vi "cRIO_FPGA_COMMUNICATION Schreibe Ausgangsdaten.vi"(8 "error in (no error)":errorcluster caption="Fehler (Eingang, kein Fehler)", 9 "Station":bool[](array[boolean])=[FALSE, FALSE, FALSE, FALSE, FALSE, FALSE, FALSE, FALSE], 10 "Band":bool[](array[boolean])=[FALSE, FALSE, FALSE, FALSE, FALSE, FALSE, FALSE, FALSE], 11 "Station Index":T1) -> (0 "error out":errorcluster caption="Fehler (Ausgang)")   [LabVIEW 2013, in "cRIO_FPGA_COMMUNICATION.lvlib"]
uses:
  cRIO_FPGA_COMMUNICATION.lvlib
  TYPES/TYPE Station Index.ctl
  TYPES/TYPE Band und Stations Kommandos.ctl
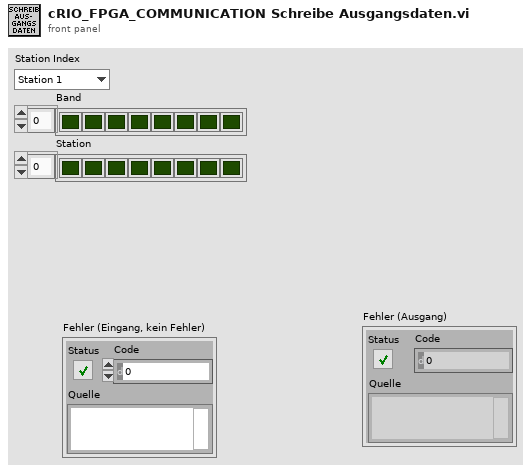
[diagram p1: front panel]
types:
  T1 = typedef "cRIO_FPGA_COMMUNICATION.lvlib/TYPE Station Index.ctl" = enum16{"Station 1", "Station 2", "Station 3", "Station 4", "Station 5", "Station 6", "Station 7", "Station 8", "Station 9", "Station 10", "Station 11", "Station 12", "Station 13", "Station 14", "Station 15", "Station 16", "Station 17", "Station 18", "Station 19", "Station 20"}
  T2 = typedef "cRIO_FPGA_COMMUNICATION.lvlib/TYPE Band und Stations Kommandos.ctl" = enum16{"Init", "Lese", "Schreibe"}
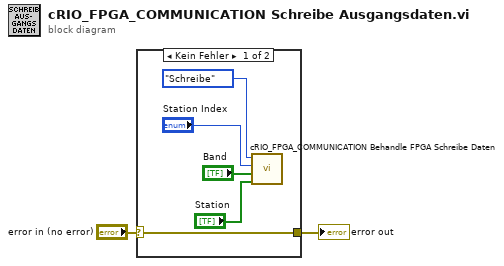
[diagram p0: block diagram]
diagram:
  n1 = case shown="Kein Fehler" "error in (no error)" {
    selector: "error in (no error)" -> [w7 w8]
    tunnel: [w7 w8] -> w1
    frame No Error {
      n2 = call "cRIO_FPGA_COMMUNICATION Behandle FPGA Schreibe Daten.vi"("Station"="Station", "Band"="Band", "Station Index"="Station Index", "FGV Band/Station Commands"=TYPE_Band_und_Stations_Kommandos."Schreibe") -> ()  [unwired: 6 in, 2 out]
    }
    frame Error {
    }
  }
  "error out" <- w1
